vi "Initialize FPGA Resources.vi"(8 "Error In":errorcluster, 11 "Audio Analyzer In":refnum<class "Audio Analyzer.lvclass">) -> (0 "Error Out":errorcluster, 3 "Audio Analyzer Out":refnum<class "Audio Analyzer.lvclass">)   [LabVIEW 2019, in "Audio Analyzer.lvclass"]
uses:
  Audio Analyzer.lvclass
  Accessors/FPGA Reference/Get FPGA Reference.vi
  <vilib>/rvi/interface/common/niFpgaWaitOnOcc.vi
  <vilib>/Utility/error.llb/Error Cluster From Error Code.vi
  Accessors/FPGA Reference/Set FPGA Reference.vi
  Public/Controls/FPGA Reference.ctl
  <vilib>/rvi/interface/nirviMethod/nirviMethod.xnode
  <vilib>/FPGAPlugInAG/Dynamic/niLvFpga_StartFifo_Dynamic.vi
  <vilib>/rvi/errors/niLvFpgaMergeErrorWithErrorCode.vi
  <vilib>/FPGAPlugInAG/Dynamic/niLvFpga_ConfigureFifo_Dynamic.vi
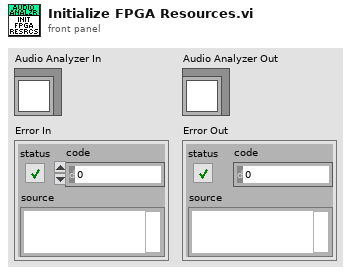
[diagram p1: front panel]
types:
  T1 = typedef "Audio Analyzer.lvclass/FPGA Reference.ctl" = refnum<k20>
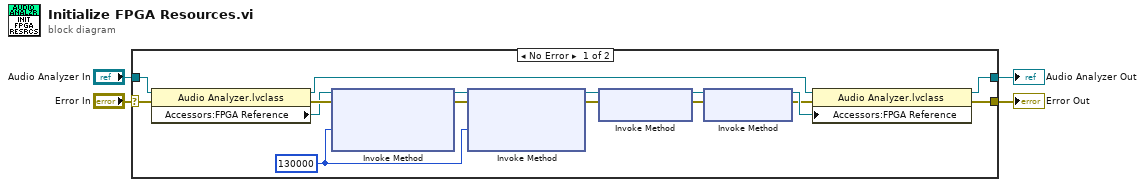
[diagram p0: block diagram]
diagram:
  n1 = case shown="No Error" "Error In" {
    selector: "Error In" -> [w13 w21]
    tunnel: [w18 w21] -> w4
    tunnel: [w17 w22] -> w3
    tunnel: "Audio Analyzer In" -> [w5 w22]
    frame No Error {
      w12 = u32 130000
      n2 = property class="Audio Analyzer.lvclass"(reference=w5, error in=w13) -> (reference out=w16:refnum<class "Audio Analyzer.lvclass">, error out=w15:errorcluster, "Accessors:FPGA Reference"=w14:T1)
      n3 = xnode "Invoke Method"("FPGA VI Reference In"=w14, "error in"=w15, "Requested Depth"=w12) -> ("FPGA VI Reference Out"=w8:T1, "error out"=w10:errorcluster)  [unwired: 1 out]
      n4 = xnode "Invoke Method"("FPGA VI Reference In"=w8, "error in"=w10, "Requested Depth"=w12) -> ("FPGA VI Reference Out"=w9:T1, "error out"=w11:errorcluster)  [unwired: 1 out]
      n5 = xnode "Invoke Method"("FPGA VI Reference In"=w9, "error in"=w11) -> ("FPGA VI Reference Out"=w6:T1, "error out"=w7:errorcluster)
      n6 = xnode "Invoke Method"("FPGA VI Reference In"=w6, "error in"=w7) -> ("FPGA VI Reference Out"=w20:T1, "error out"=w19:errorcluster)
      n7 = property class="Audio Analyzer.lvclass"(reference=w16, error in=w19, "Accessors:FPGA Reference"=w20) -> (reference out=w17:refnum<class "Audio Analyzer.lvclass">, error out=w18:errorcluster)
    }
    frame Error {
    }
  }
  "Error Out" <- w4
  "Audio Analyzer Out" <- w3
